vi "Untitled 1.vi"() -> ()   [LabVIEW 2023]
panel:
  out "XY Graph":cluster{i32[], i32[]}(graph)
  in  "Numeric":i32
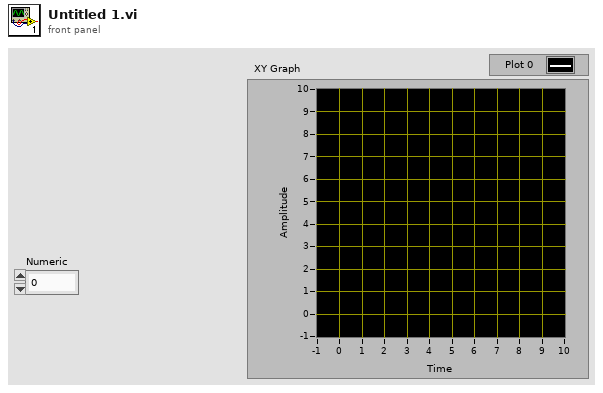
[diagram p1: front panel]
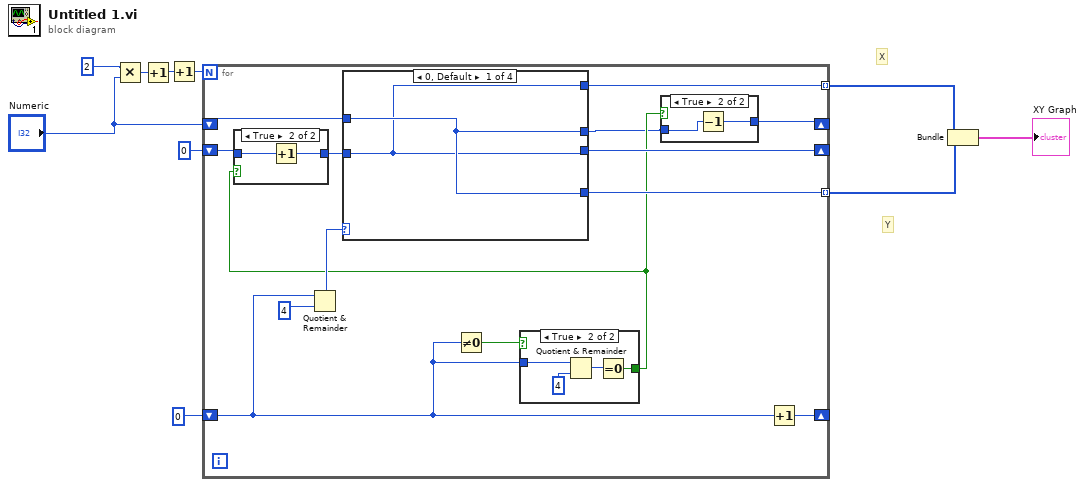
[diagram p0: block diagram]
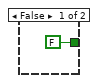
[diagram p7: hidden frame]
diagram:
  # "Y"
  # "X"
  n1 = Multiply(x=2, y="Numeric") -> (x*y=w10:i32)
  n2 = Increment(x=w10) -> (x+1=w2:i32)
  n3 = Increment(x=w2) -> (x+1=w1:i32)
  n4 = for {
    N: w1 -> [_]
    shift-right: [w11] -> _
    shift-left: "Numeric" -> [w14]
    shift-right: [w24] -> _
    shift-left: 0 -> [w21]
    tunnel: [w19] -> w6 mode=indexing
    tunnel: [w18] -> w5 mode=indexing
    shift-right: [w15] -> _
    shift-left: 0 -> [w17]
    n5 = Quotient & Remainder(x=w21, y=4) -> (x-y*floor(x/y)=w20:i32)  [unwired: 1 out]
    n6 = Not Equal To 0?(x=w21) -> (x != 0?=w23:bool)
    n7 = case shown="True" w23 {
      tunnel: w21 -> [_ w42]
      tunnel: [FALSE w40] -> w13
      frame False {
      }
      frame True {
        n8 = Quotient & Remainder(x=w42, y=4) -> (x-y*floor(x/y)=w41:i32)  [unwired: 1 out]
        n9 = Equal To 0?(x=w41) -> (x = 0?=w40:bool)
      }
    }
    n10 = case shown="True" w13 {
      tunnel: w17 -> [w28 w30]
      tunnel: [w28 w29] -> w16
      frame False {
      }
      frame True {
        n11 = Increment(x=w30) -> (x+1=w29:i32)
      }
    }
    n12 = case shown="0, Default" w20 {
      tunnel: [w32 w34 w36 w38] -> w12
      tunnel: w14 -> [w32 w34 w36 w38]
      tunnel: [w31 w33 w36 w38] -> w19
      tunnel: [w32 w33 w35 w38] -> w18
      tunnel: w16 -> [w31 w33 w35 w37]
      tunnel: [w31 w33 w35 w37] -> w15
      frame 0, Default {
      }
      frame 1 {
      }
      frame 2 {
      }
      frame 3 {
      }
    }
    n13 = case shown="True" w13 {
      tunnel: w12 -> [w25 w27]
      tunnel: [w25 w26] -> w11
      frame False {
      }
      frame True {
        n14 = Decrement(x=w27) -> (x-1=w26:i32)
      }
    }
    n15 = Increment(x=w21) -> (x+1=w24:i32)
  }
  n16 = Bundle(w6, w5) -> (→"XY Graph":cluster{i32[], i32[]})  [unwired: 1 in]
